vi "PLL analyzer -- data source -- V1.vi"(7 "data source action":T2, 9 "z  in (V)":cdb, 10 "Freq in (Hz)":dbl=40000.0 format="%#_13g", 11 "PLL data source":T1) -> (1 "z out (V)":cdb, 2 "Freq out (Hz)":dbl, 3 "PLL data source OUT":T1)   [LabVIEW 2017]
uses:
  PLL data source.ctl
  data source action.ctl
  publisher action.ctl
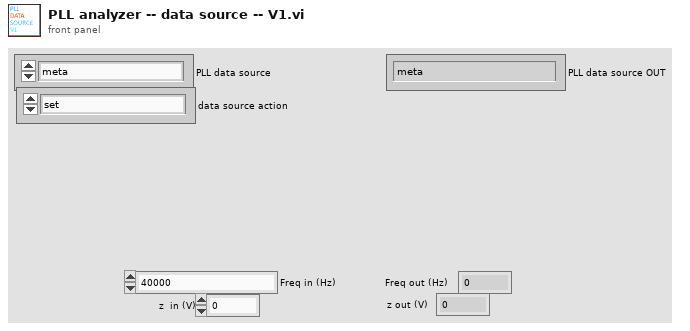
[diagram p1: front panel]
types:
  T1 = typedef "PLL data source.ctl" = enum16{"meta", "MFLI"}
  T2 = typedef "data source action.ctl" = enum16{"set", "get", "init"}
  T3 = typedef "publisher action.ctl" = enum16{"set", "get"}
  T4 = typedef "Zurich Instruments LabOne.lvlib/ziTypeHandle.ctl" = cluster{"handleValid":bool, "Conn":u64, "Path Prefix":string, "Handle":u64, "Connected":bool, "Clockbase(s)":dbl}
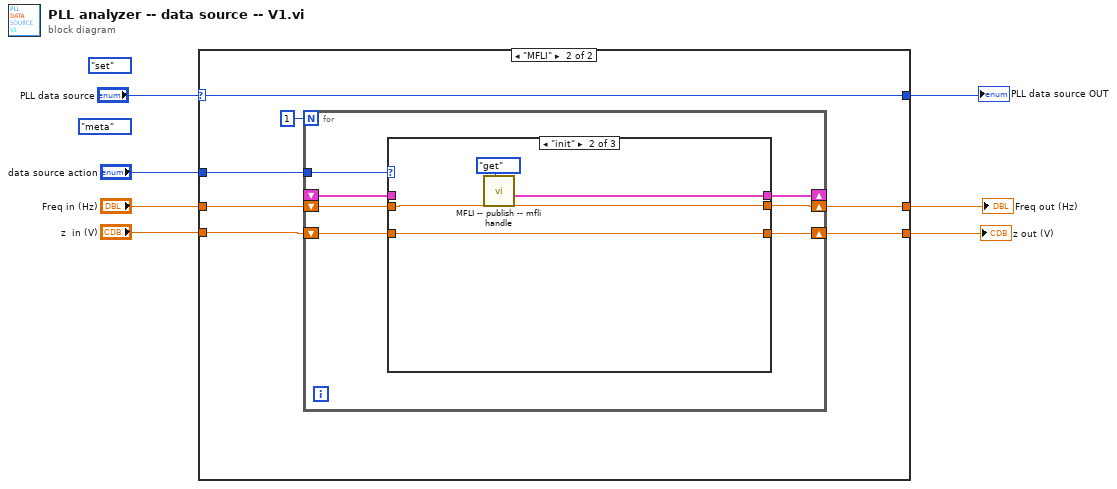
[diagram p0: block diagram]
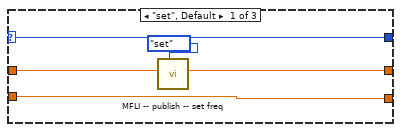
[diagram p3: hidden frame]
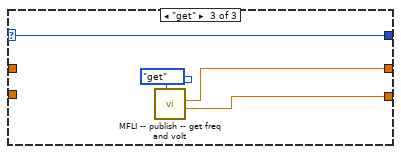
[diagram p4: hidden frame]
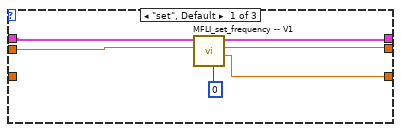
[diagram p5: hidden frame]
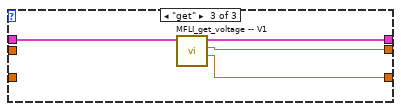
[diagram p6: hidden frame]
diagram:
  (unwired) data_source_action."set" ("data source action")
  (unwired) PLL_data_source."meta" ("PLL data source")
  n1 = case shown="\"MFLI\"" "PLL data source" {
    selector: "PLL data source" -> [w8 w27]
    tunnel: "data source action" -> [w9 w26]
    tunnel: [w12 w32] -> w5
    tunnel: [w11 w31] -> w4
    tunnel: "Freq in (Hz)" -> [w13 w30]
    tunnel: "z  in (V)" -> [w10 w29]
    tunnel: [w8 w27] -> w1
    frame "meta", Default {
      n2 = case shown="\"init\"" w9 {
        selector: w9 -> [w14 w19 w22]
        tunnel: [w16 w21 w24] -> w12
        tunnel: [w15 w20 w23] -> w11
        tunnel: w13 -> [w17 w21 _]
        tunnel: w10 -> [w15 w20 _]
        tunnel: [w14 w19 w22] -> _
        frame "set", Default {
          n3 = call "MFLI -- publish -- set freq.vi"("publisher action"=publisher_action."set", "freq IN (Hz)"=w17) -> ("freq out (Hz)"=w16:dbl)  [unwired: 9 in]
        }
        frame "init" {
        }
        frame "get" {
          n4 = call "MFLI -- publish -- get freq and volt.vi"("publisher action"=publisher_action."get") -> ("Voltage out (V)"=w23:cdb, "freq out (Hz)"=w24:dbl)  [unwired: 9 in]
        }
      }
    }
    frame "MFLI" {
      n5 = for {
        N: 1 -> [_]
        shift-right: [w39] -> _
        shift-left: _ -> [w38]
        shift-right: [w37] -> w32
        shift-left: w30 -> [w35]
        shift-right: [w36] -> w31
        shift-left: w29 -> [w34]
        tunnel: w26 -> [w33]
        n6 = case shown="\"init\"" w33 {
          tunnel: [w45 w48 w53] -> w39
          tunnel: w38 -> [w44 _ w52]
          tunnel: [w41 w46 w51] -> w37
          tunnel: [w40 w47 w50] -> w36
          tunnel: w35 -> [w42 w46 _]
          tunnel: w34 -> [_ w47 _]
          frame "set", Default {
            n7 = call "MFLI_set_frequency -- V1.vi"("Oscillator (0)"=u16 0, "Freq in (Hz)"=w42, "Handle In"=w44) -> ("z out (V)"=w40:cdb, "Freq out (Hz)"=w41:dbl, "Handle Out"=w45:T4)  [unwired: 5 in, 1 out]
          }
          frame "init" {
            n8 = call "MFLI -- publish -- mfli handle.vi"("publisher action"=publisher_action."get") -> ("Handle Out"=w48:T4)  [unwired: 10 in]
          }
          frame "get" {
            n9 = call "MFLI_get_voltage -- V1.vi"("Handle In"=w52) -> ("z out (V)"=w50:cdb, "Freq out (Hz)"=w51:dbl, "Handle Out"=w53:T4)  [unwired: 7 in, 1 out]
          }
        }
      }
    }
  }
  "Freq out (Hz)" <- w5
  "z out (V)" <- w4
  "PLL data source OUT" <- w1
